vi "check_done.vi"(11 "Mission in":refnum<class "Mission.lvclass">) -> (1 "Done?":bool, 3 "Mission out":refnum<class "Mission.lvclass">)   [LabVIEW 2011, in "Mission.lvclass"]
uses:
  Mission.lvclass
  Mission.lvclass/Mission.ctl
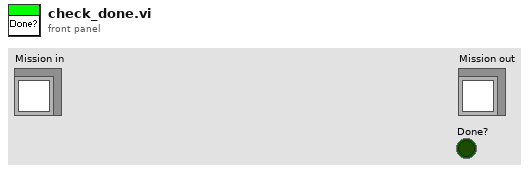
[diagram p1: front panel]
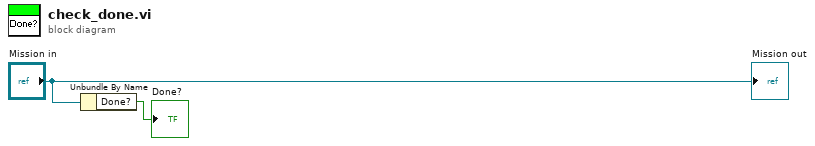
[diagram p0: block diagram]
diagram:
  n1 = Unbundle By Name("Mission in") -> ("Done?"=→"Done?":bool)
  "Mission out" <- "Mission in"
